vi "Destroy All Data Queues.vi"(8 "Error In":errorcluster, 11 "WINFAS 2 Data Queue.lvlib:All Data Queues Cluster":T1) -> (0 "Error Out":errorcluster)   [LabVIEW 2014, in "WINFAS 2 Data Queue.lvlib"]
uses:
  WINFAS 2 Data Queue.lvlib
  All Data Queues Cluster.ctl
  Acquisition Data 1 Sample Cluster.ctl
  Control Data Cluster.ctl
  Async Acquisition Data Cluster.ctl
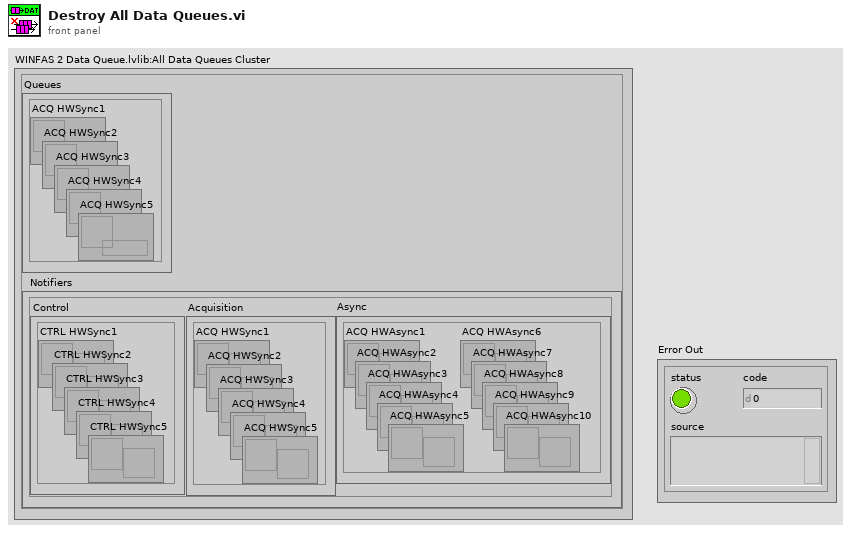
[diagram p1: front panel]
types:
  T1 = typedef "WINFAS 2 Data Queue.lvlib/All Data Queues Cluster.ctl" = cluster{"Queues":cluster{"ACQ HWSync1":refnum<queue>, "ACQ HWSync2":refnum<queue>, "ACQ HWSync3":refnum<queue>, "ACQ HWSync4":refnum<queue>, "ACQ HWSync5":refnum<queue>}, "Notifiers":cluster{"Control":cluster{"CTRL HWSync1":refnum<notifier>, "CTRL HWSync2":refnum<notifier>, "CTRL HWSync3":refnum<notifier>, "CTRL HWSync4":refnum<notifier>, "CTRL HWSync5":refnum<notifier>}, "Acquisition":cluster{"ACQ HWSync1":refnum<notifier>, "ACQ HWSync2":refnum<notifier>, "ACQ HWSync3":refnum<notifier>, "ACQ HWSync4":refnum<notifier>, "ACQ HWSync5":refnum<notifier>}, "Async":cluster{"ACQ HWAsync1":refnum<notifier>, "ACQ HWAsync2":refnum<notifier>, "ACQ HWAsync3":refnum<notifier>, "ACQ HWAsync4":refnum<notifier>, "ACQ HWAsync5":refnum<notifier>, "ACQ HWAsync6":refnum<notifier>, "ACQ HWAsync7":refnum<notifier>, "ACQ HWAsync8":refnum<notifier>, "ACQ HWAsync9":refnum<notifier>, "ACQ HWAsync10":refnum<notifier>}}}
  T2 = cluster{"ACQ HWSync1":refnum<queue>, "ACQ HWSync2":refnum<queue>, "ACQ HWSync3":refnum<queue>, "ACQ HWSync4":refnum<queue>, "ACQ HWSync5":refnum<queue>}
  T3 = cluster{"Control":cluster{"CTRL HWSync1":refnum<notifier>, "CTRL HWSync2":refnum<notifier>, "CTRL HWSync3":refnum<notifier>, "CTRL HWSync4":refnum<notifier>, "CTRL HWSync5":refnum<notifier>}, "Acquisition":cluster{"ACQ HWSync1":refnum<notifier>, "ACQ HWSync2":refnum<notifier>, "ACQ HWSync3":refnum<notifier>, "ACQ HWSync4":refnum<notifier>, "ACQ HWSync5":refnum<notifier>}, "Async":cluster{"ACQ HWAsync1":refnum<notifier>, "ACQ HWAsync2":refnum<notifier>, "ACQ HWAsync3":refnum<notifier>, "ACQ HWAsync4":refnum<notifier>, "ACQ HWAsync5":refnum<notifier>, "ACQ HWAsync6":refnum<notifier>, "ACQ HWAsync7":refnum<notifier>, "ACQ HWAsync8":refnum<notifier>, "ACQ HWAsync9":refnum<notifier>, "ACQ HWAsync10":refnum<notifier>}}
  T4 = cluster{"CTRL HWSync1":refnum<notifier>, "CTRL HWSync2":refnum<notifier>, "CTRL HWSync3":refnum<notifier>, "CTRL HWSync4":refnum<notifier>, "CTRL HWSync5":refnum<notifier>}
  T5 = cluster{"ACQ HWSync1":refnum<notifier>, "ACQ HWSync2":refnum<notifier>, "ACQ HWSync3":refnum<notifier>, "ACQ HWSync4":refnum<notifier>, "ACQ HWSync5":refnum<notifier>}
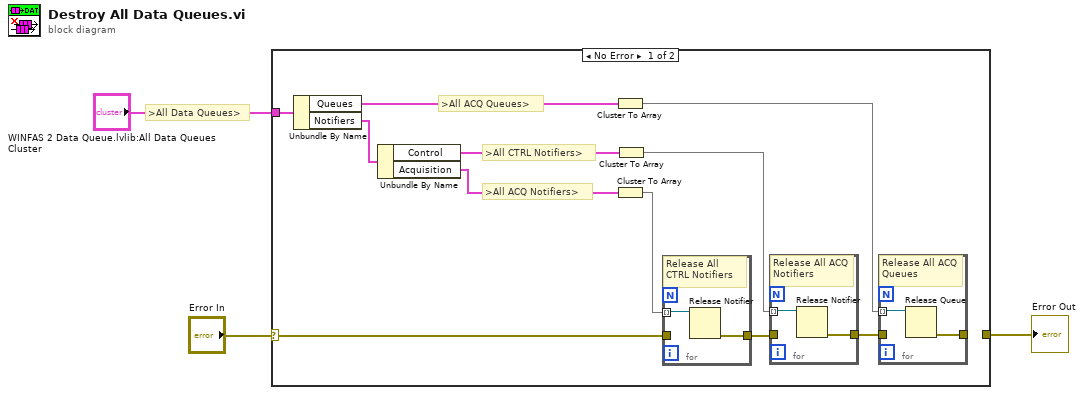
[diagram p0: block diagram]
diagram:
  # ">All Data Queues>"
  n1 = case shown="No Error" "Error In" {
    selector: "Error In" -> [w11 w21]
    tunnel: [_ w21] -> w2
    tunnel: "WINFAS 2 Data Queue.lvlib:All Data Queues Cluster" -> [w14 _]
    frame No Error {
      # ">All ACQ Notifiers>"
      # ">All CTRL Notifiers>"
      # ">All ACQ Queues>"
      n2 = Unbundle By Name(w14) -> ("Queues"=w13:T2, "Notifiers"=w6:T3)
      n3 = Unbundle By Name(w6) -> ("Control"=w4:T4, "Acquisition"=w5:T5)
      n4 = Cluster To Array(cluster=w13) -> (array=w7:refnum<queue>[])
      n5 = Cluster To Array(cluster=w5) -> (array=w12:refnum<notifier>[])
      n6 = Cluster To Array(cluster=w4) -> (array=w8:refnum<notifier>[])
      n7 = for {
        tunnel: w12 -> [w20] mode=indexing
        tunnel: w11 -> [_]
        tunnel: [w19] -> w10
        # "Release All CTRL Notifiers"
        n8 = Release Notifier(notifier=w20) -> (error out=w19:errorcluster)  [unwired: 2 in, 2 out]
      }
      n9 = for {
        tunnel: w8 -> [w18] mode=indexing
        tunnel: w10 -> [_]
        tunnel: [w17] -> w9
        # "Release All ACQ Notifiers"
        n10 = Release Notifier(notifier=w18) -> (error out=w17:errorcluster)  [unwired: 2 in, 2 out]
      }
      n11 = for {
        tunnel: w7 -> [w16] mode=indexing
        tunnel: w9 -> [_]
        tunnel: [w15] -> _
        # "Release All ACQ Queues"
        n12 = Release Queue(queue=w16) -> (error out=w15:errorcluster)  [unwired: 2 in, 2 out]
      }
    }
    frame Error {
    }
  }
  "Error Out" <- w2
